vi "Arrival_time_weighting_1.vi"(1 "Arrival times":dbl[](array[numeric]) format="%.2f") -> (0 "Weighting":dbl[](array[numeric]) format="%.2f")   [LabVIEW 2011]
panel:
  out "int arrival time":dbl[](array[numeric])
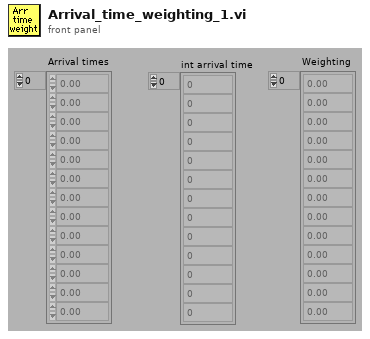
[diagram p1: front panel]
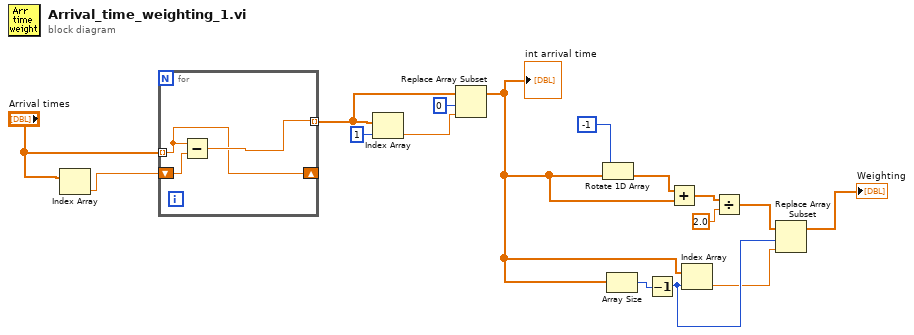
[diagram p0: block diagram]
diagram:
  n1 = Index Array(array="Arrival times") -> (element=w15:dbl)  [unwired: 1 in]
  n2 = for {
    shift-right: [w17] -> _
    shift-left: w15 -> [w19]
    tunnel: "Arrival times" -> [w17] mode=indexing
    tunnel: [w18] -> w13 mode=indexing
    n3 = Subtract(x=w17, y=w19) -> (x-y=w18:dbl)
  }
  n4 = Index Array(array=w13, index=1) -> (element=w11:dbl)
  n5 = Replace Array Subset(array=w13, new element=w11, index=0) -> (w5:dbl[])
  "int arrival time" <- w5
  n6 = Rotate 1D Array(1:w5, 2:-1 ("n")) -> (0:w7:dbl[])
  n7 = Array Size(array=w5) -> (size(s)=w6:i32)
  n8 = Decrement(x=w6) -> (x-1=w2:i32)
  n9 = Add(x=w7, y=w5) -> (x+y=w9:dbl[])
  n10 = Index Array(array=w5, index=w2) -> (element=w1:dbl)
  n11 = Divide(x=w9, y=2.0) -> (x/y=w4:dbl[])
  n12 = Replace Array Subset(array=w4, new element=w1, index=w2) -> (→"Weighting":dbl[])
